vi "Relative Sound Files.vi"() -> ()   [LabVIEW 2009]
panel:
  out "temperaturelimit":string
  out "xpexcl":string
  out "xpnotify":string
  out "xperror":string
  out "xpding":string
  out "critstop":string
  out "battlow":string
  out "battcrit":string
  out "tada":string
  out "notify":string
  out "chord":string
  out "ding":string
  out "startup":string
  out "goodbye":string
  out "train":string
  out "terminated":string
  out "notready":string
  out "scanint":string
  out "scancancel":string
  out "error":string
  out "scanbelong":string
  out "PClimit":string
  out "pause":string
  out "lowcryo":string
  out "danger":string
  out "allscans":string
  out "scandone":string
  out "sweepint":string
  out "leavepersis":string
  out "enterpersis":string
  out "zero":string
  out "field":string
  out "lvlN":string
  out "lvlHe":string
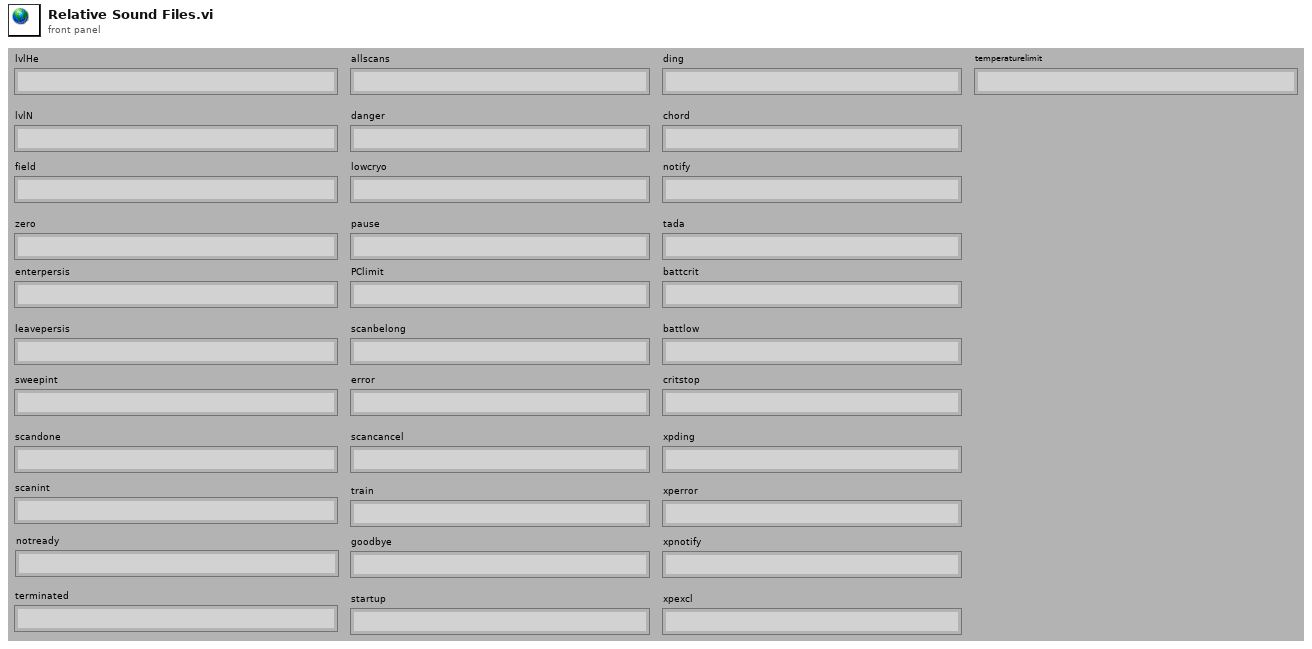
[diagram p1: front panel]
diagram:
